vi "GET Input Voltage Limits.vi"() -> (0 "Maximum Input Voltage":dbl, 1 "Minimum Input Voltage":dbl)   [LabVIEW 2013]
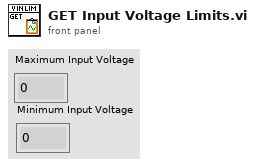
[diagram p1: front panel]
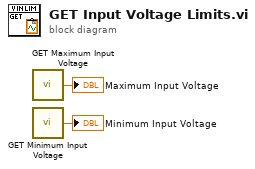
[diagram p0: block diagram]
diagram:
  n1 = call "GET Maximum Input Voltage.vi"() -> ("Maximum Input Voltage"=→"Maximum Input Voltage":dbl)
  n2 = call "GET Minimum Input Voltage.vi"() -> ("Minimum Input Voltage"=→"Minimum Input Voltage":dbl)
